vi "acknowledge Over Pressure.vi"(8 "error in (no error)":errorcluster, 10 "channel":u32, 11 "pumpIndex":u32) -> (0 "error out":errorcluster, 3 "function return":i32)   [LabVIEW 2018, in "AsiaPumpInterface.lvlib"]
doc: "extern ASIAPUMP_INTERFACE_API BOOL acknowledgeOverPressure( unsigned int pumpIndex ,\n unsigned int channel );"
uses:
  <userlib>/AsiaPumpInterface/AsiaPumpInterface.lvlib
  <userlib>/AsiaPumpInterface/AsiaPumpInterface.dll
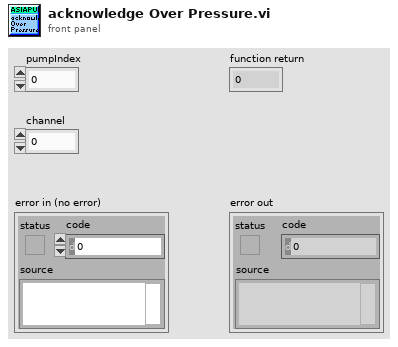
[diagram p1: front panel]
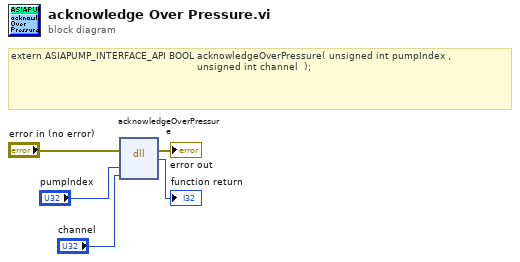
[diagram p0: block diagram]
diagram:
  # "extern ASIAPUMP_INTERFACE_API BOOL acknowledgeOverPressure( unsigned int pumpIndex ,\n                                                              unsigned int channel  );"
  n1 = dll-call lib="C:/Program Files (x86)/National Instruments/LabVIEW 2018/user.lib/AsiaPumpInterface/AsiaPumpInterface.*" fn="acknowledgeOverPressure"(error in="error in (no error)", "pumpIndex"="pumpIndex", "channel"="channel") -> (error out=→"error out":errorcluster, →"function return":i32)  [unwired: 4 in, 1 out]
